vi "Event Driven State Machine Template.vi"() -> ()   [LabVIEW 2014]
panel:
  in  "Run Button":bool
  in  "Process Stop Button":bool
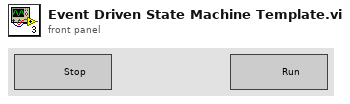
[diagram p1: front panel]
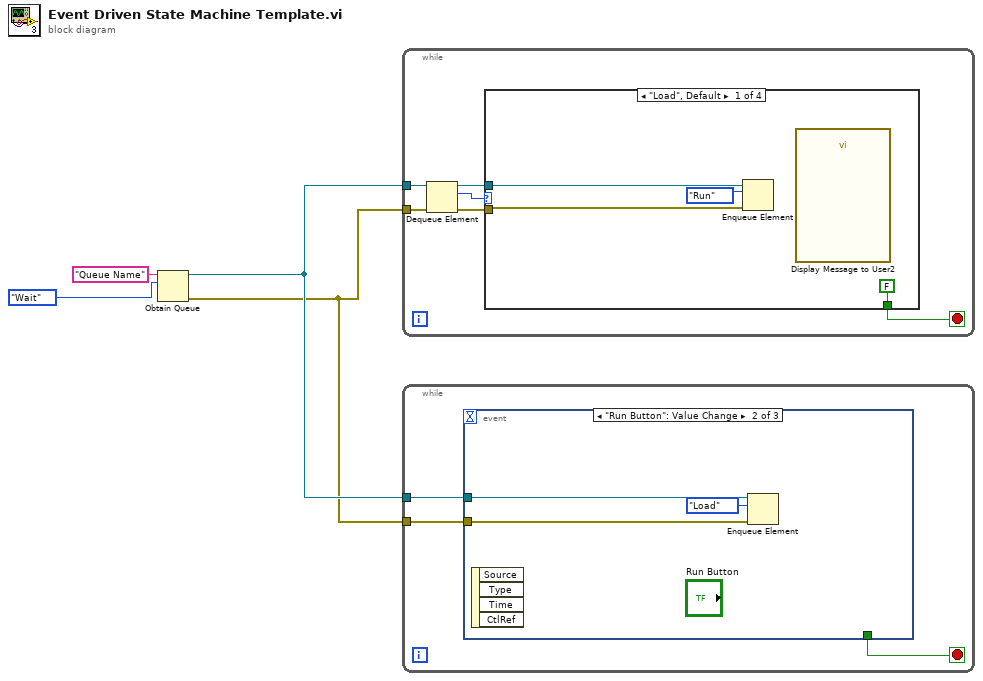
[diagram p0: block diagram]
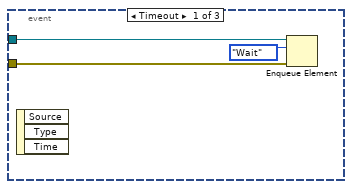
[diagram p2: hidden frame]
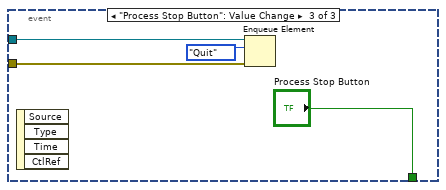
[diagram p3: hidden frame]
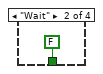
[diagram p4: hidden frame]
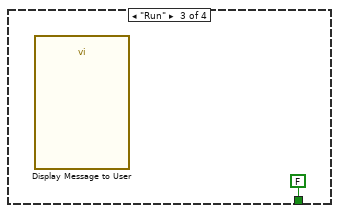
[diagram p5: hidden frame]
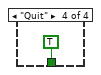
[diagram p6: hidden frame]
diagram:
  n1 = Obtain Queue(name (unnamed)="Queue Name", element data type=enum16{"Load", "Wait", "Run", "Quit"}."Wait") -> (queue out=w3:refnum<queue>, error out=w1:errorcluster)  [unwired: 3 in, 1 out]
  n2 = while {
    tunnel: w3 -> [w10]
    tunnel: w1 -> [w9]
    stop <- w5 stop-if-true
    n3 = Dequeue Element(queue=w10, error in (no error)=w9) -> (queue out=w7:refnum<queue>, element=w8:enum16{"Load", "Wait", "Run", "Quit"}, error out=w6:errorcluster)  [unwired: 1 in, 1 out]
    n4 = case shown="\"Load\", Default" w8 {
      tunnel: w7 -> [w14 _ _ _]
      tunnel: w6 -> [w13 _ _ _]
      tunnel: [FALSE FALSE FALSE TRUE] -> w5
      frame "Load", Default {
        n5 = Enqueue Element(queue=w14, element=enum16{"Load", "Wait", "Run", "Quit"}."Run", error in (no error)=w13) -> ()  [unwired: 1 in, 3 out]
        n6 = call "Display Message to User2"() -> ()  [unwired: 10 in, 2 out]
      }
      frame "Wait" {
      }
      frame "Run" {
        n7 = call "Display Message to User"() -> ()  [unwired: 10 in, 2 out]
      }
      frame "Quit" {
      }
    }
  }
  n8 = while {
    tunnel: w3 -> [w20]
    tunnel: w1 -> [w19]
    stop <- w18 stop-if-true
    n9 = event shown="[1] \"Run Button\": Value Change" {
      selector: _ -> [_ _ _]
      dyn-events: _ -> [_ _ _]
      timeout: _ -> [_ _ _]
      tunnel: w20 -> [w23 w26 w30]
      tunnel: w19 -> [w22 w25 w29]
      tunnel: [_ _ "Process Stop Button"] -> w18
      event Timeout {
        n10 = event-data() -> ()  [unwired: 1 in, 3 out]
        n11 = Enqueue Element(queue=w23, element=enum16{"Load", "Wait", "Run", "Quit"}."Wait", error in (no error)=w22) -> ()  [unwired: 1 in, 3 out]
      }
      event "Run Button": Value Change {
        n12 = event-data() -> ()  [unwired: 1 in, 4 out]
        n13 = Enqueue Element(queue=w26, element=enum16{"Load", "Wait", "Run", "Quit"}."Load", error in (no error)=w25) -> ()  [unwired: 1 in, 3 out]
      }
      event "Process Stop Button": Value Change {
        n14 = event-data() -> ()  [unwired: 1 in, 4 out]
        n15 = Enqueue Element(queue=w30, element=enum16{"Load", "Wait", "Run", "Quit"}."Quit", error in (no error)=w29) -> ()  [unwired: 1 in, 3 out]
      }
    }
  }
